vi "Digio Read Bit.vi"(7 "Bit (1)":u32=1 min=1 max=14, 8 "error in (no error)":errorcluster, 10 "Node In":string, 11 "VISA resource name":refnum<visa-resource-name>) -> (0 "error out":errorcluster, 1 "Data":i32, 2 "Node Out":string, 3 "VISA resource name out":refnum<visa-resource-name>, 4 "Command String":string)   [LabVIEW 2018, in "Keithley 2600 Series.lvlib"]
doc: "This VI will read one digital I/O line.\n\n<b>Functions and Attributes Used</b>\ndigio.readbit(bit)\nbit = Digital I/O line number to be read (1 to 14)\n\nNote:\nDigital IO feature is not supported with Keithley 2604B, 2614B, 2634B."
uses:
  Keithley 2600 Series.lvlib
  Private/GlobalVariables.vi
panel:
  # "(c) 2008 Keithley Instruments, Inc.  ALL RIGHTS RESERVED."
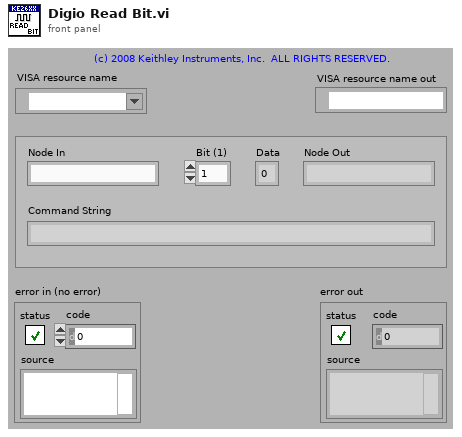
[diagram p1: front panel]
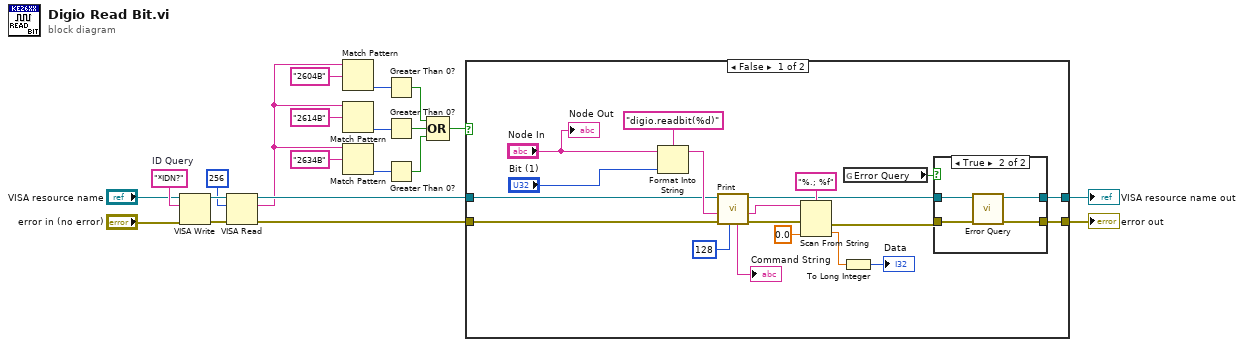
[diagram p0: block diagram]
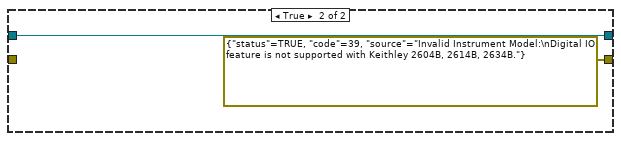
[diagram p3: hidden frame]
diagram:
  w16 = "*IDN?"  # ID Query
  n1 = VISA Write(VISA resource name="VISA resource name", write buffer=w16, error in (no error)="error in (no error)") -> (VISA resource name out=w19:refnum<visa-resource-name>, error out=w18:errorcluster)  [unwired: 1 out]
  n2 = VISA Read(VISA resource name=w19, byte count=u32 256, error in (no error)=w18) -> (VISA resource name out=w15:refnum<visa-resource-name>, read buffer=w1:string, error out=w14:errorcluster)  [unwired: 1 out]
  n3 = Match Pattern(string=w1, regular expression="2604B" ("y")) -> (offset past match=w8:i32)  [unwired: 1 in, 3 out]
  n4 = Match Pattern(string=w1, regular expression="2614B" ("y")) -> (offset past match=w7:i32)  [unwired: 1 in, 3 out]
  n5 = Match Pattern(string=w1, regular expression="2634B" ("y")) -> (offset past match=w6:i32)  [unwired: 1 in, 3 out]
  n6 = Greater Than 0?(x=w8) -> (x > 0?=w5:bool)
  n7 = Greater Than 0?(x=w7) -> (x > 0?=w4:bool)
  n8 = Greater Than 0?(x=w6) -> (x > 0?=w3:bool)
  n9 = Compound Arithmetic op=OR(w5, w4, w3) -> (w2:bool)
  n10 = case shown="False" w2 {
    tunnel: [w34 w48] -> w21
    tunnel: [w33 errorcluster {"status"=TRUE, "code"=39, "source"="Invalid Instrument Model:\nDigital IO feature is not supported with Keithley 2604B, 2614B, 2634B."} ("error out")] -> w20
    tunnel: w15 -> [w23 w48]
    tunnel: w14 -> [w22 _]
    frame False {
      n11 = Format Into String(format string="digio.readbit(%d)", initial string="Node In", "Bit (1)") -> (resulting string=w26:string)  [unwired: 1 in, 1 out]
      n12 = call "Print.vi"("Byte Count (1024)"=u32 128, "error in (no error)"=w22, "Input"=w26, "VISA resource name"=w23) -> ("error out"=w28:errorcluster, "Output"=w27:string, "VISA resource name out"=w29:refnum<visa-resource-name>, "Command String"=→"Command String":string)  [unwired: 1 in, 3 out]
      n13 = Scan From String(format string="%.; %f", input string=w27, error in=w28, default 1=0.0 ("default value 1")) -> (error out=w35:errorcluster, output 1=w37:dbl)  [unwired: 1 in, 2 out]
      n14 = To Long Integer(number=w37) -> (32bit integer=→"Data":i32)
      n15 = global read "GlobalVariables.vi" "Error Query"() -> (w36:bool)
      n16 = case shown="True" w36 {
        tunnel: w29 -> [w42 w46]
        tunnel: w35 -> [w41 w45]
        tunnel: [w42 w44] -> w34
        tunnel: [w41 w43] -> w33
        frame False {
        }
        frame True {
          n17 = call "Error Query.vi"("error in (no error)"=w45, "VISA resource name"=w46) -> ("error out"=w43:errorcluster, "VISA resource name out"=w44:refnum<visa-resource-name>)  [unwired: 8 out]
        }
      }
      "Node Out" <- "Node In"
    }
    frame True {
    }
  }
  "VISA resource name out" <- w21
  "error out" <- w20
